vi "uActor_Exec.vi"(6 "Original uMsg":refnum<class "uMsg.lvclass">, 8 "error in (no error)":errorcluster, 9 "Data":refnum<class "uData.lvclass">, 10 "Command":string, 11 "Test_uActor_StreamingSubscriber in":refnum<class "Test_uActor_StreamingSubscriber.lvclass">) -> (0 "error out":errorcluster, 1 "reply":refnum<class "uData.lvclass">, 3 "Test_uActor_StreamingSubscribe out":refnum<class "Test_uActor_StreamingSubscriber.lvclass">)   [LabVIEW 2021, in "Test_uActor_StreamingSubscriber.lvclass"]
doc: "Dynamic dispatch method to allow children actors to handle incoming string commands.\n\nThe parent method returns an error if it receives an unknown incoming command."
uses:
  Test_uActor_StreamingSubscriber.lvclass
  Bin/uData.lvlibp/uData.lvclass
  Bin/uFramework.lvlibp/uMsg/uMsg.lvclass
  1e7f0096-a9c0-4b6d-b2b7-534433df7a4b.vi
  Bin/uData.lvlibp/Get Tag.vi
  Bin/uFramework.lvlibp/uActor/uActor.lvclass
  U:/Projects/uFramework/Bin/uFramework.lvlibp/uActor/uActor.lvclass
panel:
  out "i (A)":i32
  out "Latency (ms) A":u32
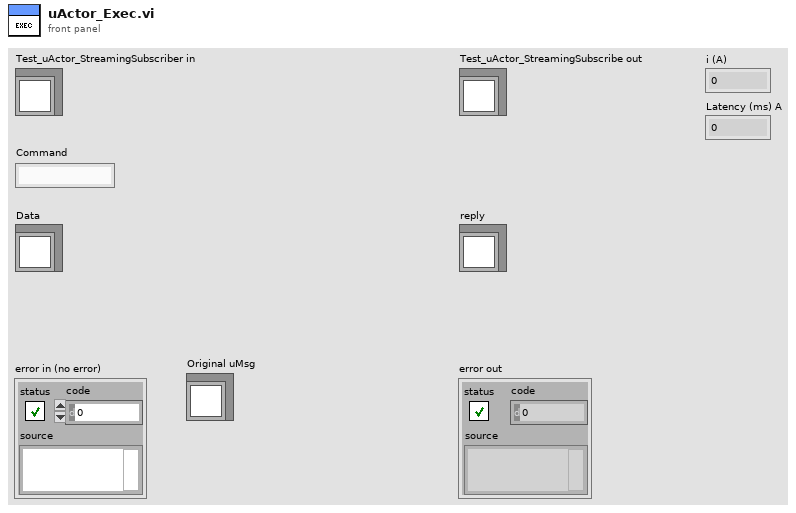
[diagram p1: front panel]
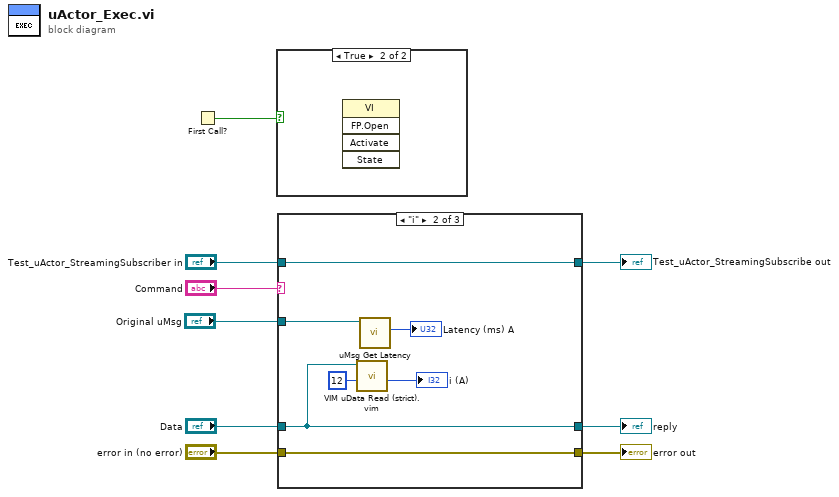
[diagram p0: block diagram]
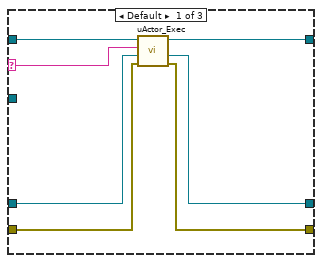
[diagram p3: hidden frame]
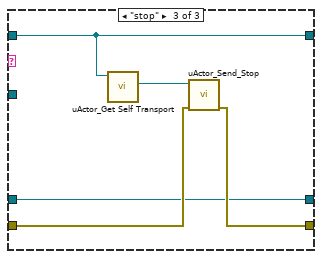
[diagram p4: hidden frame]
diagram:
  n1 = First Call?() -> (First Call?: T/F=w4:bool)
  n2 = case shown="True" w4 {
    frame False {
    }
    frame True {
      n3 = invoke class="VI" method="FP.Open"() -> ()  [unwired: 5 in, 5 out]
    }
  }
  n4 = case shown="\"i\"" "Command" {
    selector: "Command" -> [w10 _ _]
    tunnel: [w16 w20 w24] -> w9
    tunnel: [w15 w23 w28] -> w2
    tunnel: "Data" -> [w14 w20 w24]
    tunnel: "Test_uActor_StreamingSubscriber in" -> [w13 w23 w28]
    tunnel: "error in (no error)" -> [w12 w22 w26]
    tunnel: [w11 w22 w25] -> w6
    tunnel: "Original uMsg" -> [_ w19 _]
    frame Default {
      n5 = call-parent "uActor_Exec.vi"("error in (no error)"=w12, "Data"=w14, "Command"=w10, "uActor in"=w13) -> ("error out"=w11:errorcluster, "reply"=w16:refnum<class "uData.lvclass">, "uActor out"=w15:refnum<class "Test_uActor_StreamingSubscriber.lvclass">)  [unwired: 5 in]
    }
    frame "i" {
      n6 = call "VIM uData Read (strict).vim"("default value"=u32 12 ("Latency (ms) A"), "uData in"=w20) -> ("value"=→"i (A)":u32)  [unwired: 6 in, 3 out]
      n7 = call "uMsg Get Latency.vi"("uMsg in"=w19) -> ("Latency (ms)"=→"Latency (ms) A":u32)  [unwired: 8 in, 2 out]
    }
    frame "stop" {
      n8 = call "uActor_Get Self Transport.vi"("uActor in"=w28) -> ("Actor Transport"=w27:refnum<class "uTransport_uActor.lvclass">)  [unwired: 9 in, 1 out]
      n9 = call "uActor_Send_Stop.vi"("error in (no error)"=w26, "uActor Transport"=w27) -> ("error out"=w25:errorcluster)  [unwired: 9 in]
    }
  }
  "error out" <- w6
  "reply" <- w9
  "Test_uActor_StreamingSubscribe out" <- w2
